vi "Data Handler Example.vi"(8 "error in (no error)":errorcluster) -> (0 "error out":errorcluster)   [LabVIEW 2010]
panel:
  out "Sum":dbl
  in  "Enum":enum16{"Measure", "Read", "Clear Buffer"}(ring)
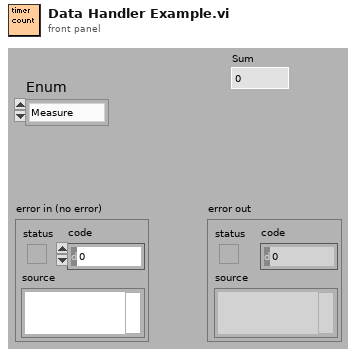
[diagram p1: front panel]
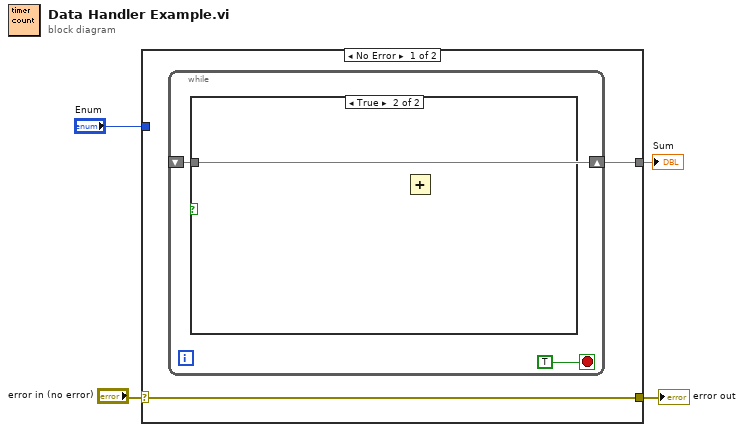
[diagram p0: block diagram]
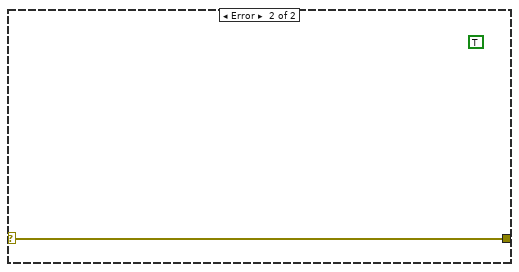
[diagram p3: hidden frame]
diagram:
  n1 = case shown="No Error" "error in (no error)" {
    selector: "error in (no error)" -> [w7 w10]
    tunnel: [w7 w10] -> w3
    tunnel: "Enum" -> [w6 _]
    tunnel: [w5 _] -> w1
    frame No Error {
      n2 = while {
        shift-right: [w8] -> w5
        shift-left: _ -> [w8]
        stop <- TRUE stop-if-true
        n3 = case shown="True" {
          selector: _ -> [_ _]
          tunnel: w8 -> [_ _]
          frame False {
          }
          frame True {
            n4 = Add() -> ()  [unwired: 2 in, 1 out]
          }
        }
      }
    }
    frame Error {
      (unwired) TRUE
    }
  }
  "error out" <- w3
  "Sum" <- w1
